vi "CustomBeep.vi"(1 "Frequency":dbl=500.0, 2 "Approx Duration (ms)":i32=5) -> ()   [LabVIEW 2022 SP3]
uses:
  <vilib>/sound2/lvsound2.llb/Sampling Mode.ctl
  <vilib>/sound2/lvsound2.llb/Sound Data Format.ctl
  <vilib>/sound2/lvsound2.llb/Sound Output Set Volume (Single).vi
  <vilib>/sound2/lvsound2.llb/Sound Output Write (DBL Single).vi
panel:
  out "Actual Length (ms)":u32
  in  "Device ID":u32
  in  "Stop":bool
  out "Generated Sound":waveform(dbl)(graph)
  in  "Volume":dbl(slide)=50.0 scale=0.0..100.0
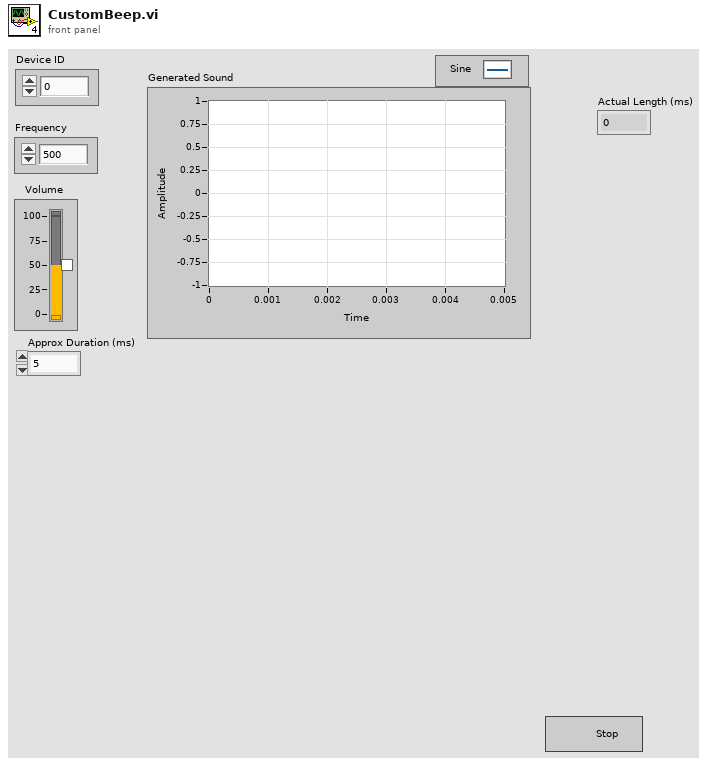
[diagram p1: front panel]
types:
  T1 = typedef "Sound Data Format.ctl" = cluster{"sample rate (S/s)":dbl, "number of channels":i32, "bits per sample":i32}
  T2 = typedef "Sampling Mode.ctl" = i32
  T3 = typedef "Sound Output Task ID.ctl" = u32
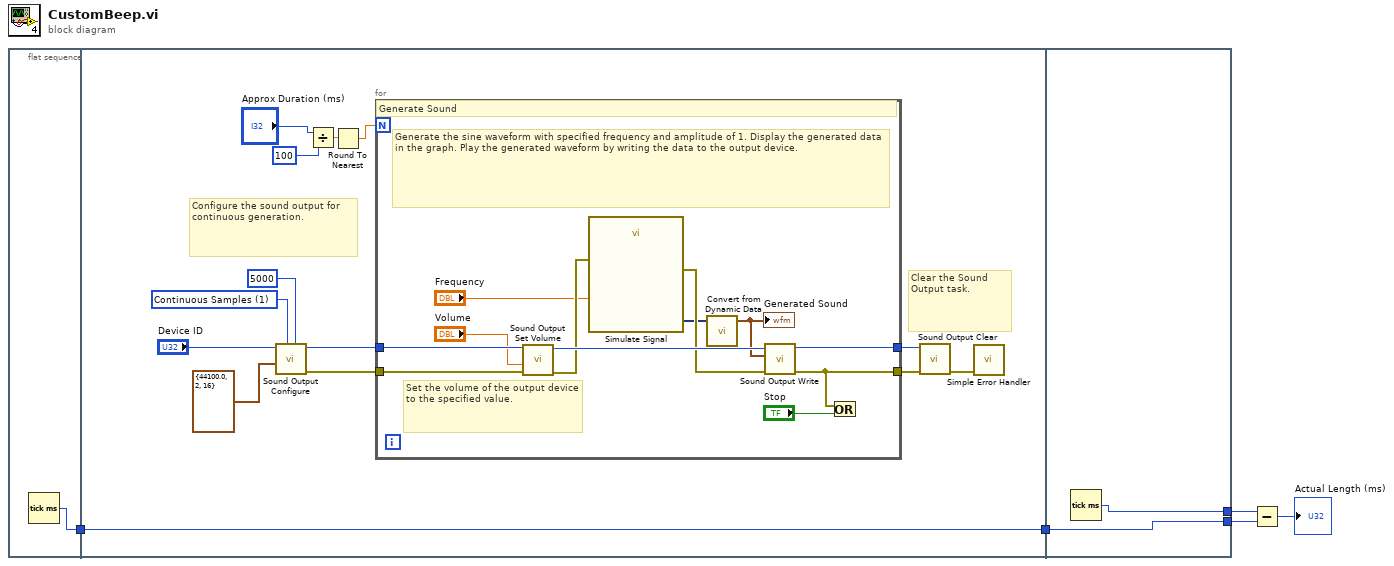
[diagram p0: block diagram]
diagram:
  n1 = flat-sequence {
    tunnel: [w6] -> w3
    tunnel: [w11] -> w4
    tunnel: w3 -> [w11]
    tunnel: [w34] -> w5
    tunnel: w4 -> [w33]
    tunnel: [w33] -> w2
    frame #0 {
      n2 = Tick Count (ms)() -> (millisecond timer value=w6:u32)
    }
    frame #1 {
      w15 = T2 1 items=["Finite Samples", "Continuous Samples"] ("sample mode")
      # "Configure the sound output for continuous generation."
      # "Clear the Sound Output task."
      n3 = call <vilib>:"Sound Output Configure.vi"("number of samples/ch"=5000 ("Number of Samples/ch"), "sample mode"=w15, "sound format"=T1 {"sample rate (S/s)"=44100.0, "number of channels"=2, "bits per sample"=16} ("Sound Format"), "device ID"="Device ID") -> ("error out"=w20:errorcluster, "task ID"=w19:T3)  [unwired: 6 in]
      n4 = Divide(x="Approx Duration (ms)", y=100) -> (x/y=w8:dbl)
      n5 = Round To Nearest(number=w8) -> (nearest integer value=w7:dbl)
      n6 = for {
        N: w7 -> [_]
        tunnel: w19 -> [w28]
        tunnel: [w32] -> w17
        tunnel: w20 -> [w30]
        tunnel: [w26] -> w18
        # "Set the volume of the output device to the specified value."
        # "Generate the sine waveform with specified frequency and amplitude of 1. Display the generated data in the graph. Play the generated waveform by writing the data to the output device."
        # "Generate Sound"
        n7 = call-poly <vilib>:"Sound Output Set Volume.vi"("error in (no error)"=w30, "volume"="Volume", "task ID"=w28) -> ("error out"=w24:errorcluster, "task ID out"=w29:T3)  [unwired: 7 in]
        n8 = call "Simulate Signal"("Frequency"="Frequency", "error in (no error)"=w24) -> ("Sine"=w22:dynamicdata, "error out"=w23:errorcluster)  [unwired: 12 in]
        n9 = call "Convert from Dynamic Data"("Dynamic Data Type"=w22) -> ("Waveform"=w25:waveform(dbl))  [unwired: 3 in]
        "Generated Sound" <- w25
        n10 = call-poly <vilib>:"Sound Output Write.vi"("error in (no error)"=w23, "data"=w25, "task ID"=w29) -> ("error out"=w26:errorcluster, "task ID out"=w32:T3)  [unwired: 7 in]
        n11 = Or(x=w26, y="Stop") -> ()  [unwired: 1 out]
      }
      n12 = call <vilib>:"Sound Output Clear.vi"("error in (no error)"=w18, "task ID"=w17) -> ("error out"=w13:errorcluster)  [unwired: 9 in]
      n13 = call <vilib>:"Simple Error Handler.vi"("error in (no error)"=w13) -> ()  [unwired: 4 in, 5 out]
    }
    frame #2 {
      n14 = Tick Count (ms)() -> (millisecond timer value=w34:u32)
    }
  }
  n15 = Subtract(x=w5, y=w2) -> (x-y=→"Actual Length (ms)":u32)
